vi "RemoveHintCallback.vi"(8 "No Error":errorcluster, 9 "Userdata [void *]":i64, 10 "Callback [SDL_HintCallback]":i64, 11 "Hint Name":T1) -> (0 "error out":errorcluster)   [LabVIEW 2024, in "SDL3.lvlib" / "Hints.lvlib"]
doc: "<B>LabVIEW Dev Note</B>\nI don't know why <B>Callback</B> and <B>Userdata</B> input are required... makes no sense...\n\n<B>Summary</B>\nRemove a function watching a particular hint."
uses:
  Hints.lvlib
  Lib/SDL3.dll
  HintName--combobox.ctl
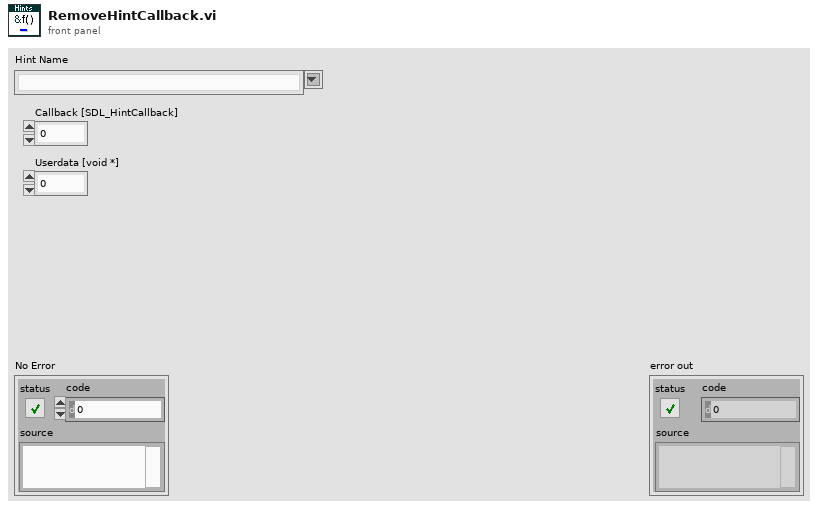
[diagram p1: front panel]
types:
  T1 = typedef "SDL3.lvlib/Hints.lvlib/HintName--combobox.ctl" = string
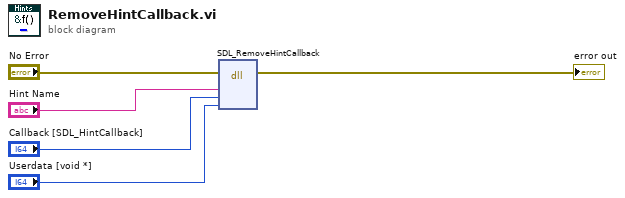
[diagram p0: block diagram]
diagram:
  n1 = dll-call lib="C:/Users/Thomas/Documents/Projects/LV-SDL3/Sources/SDL3/Lib/SDL3.*" fn="SDL_RemoveHintCallback"(error in="No Error", "name"="Hint Name", "callback"="Callback [SDL_HintCallback]", "userdata"="Userdata [void *]") -> (error out=→"error out":errorcluster)  [unwired: 6 in, 1 out]
